vi "UIRef.vi"(8 "error in":errorcluster, 11 "PXI in":refnum<class "PLTarget PXI.lvclass">) -> (0 "error out":errorcluster, 2 "VI refnum":refnum<vi>, 3 "PXI out":refnum<class "PLTarget PXI.lvclass">)   [LabVIEW 2013, in "PLTarget PXI.lvclass"]
uses:
  PLTarget PXI.lvclass
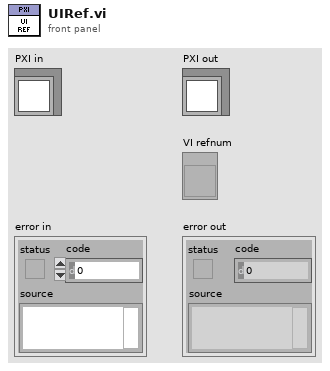
[diagram p1: front panel]
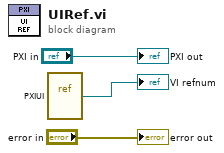
[diagram p0: block diagram]
diagram:
  n1 = vi-ref "PXIUI.vi"() -> (→"VI refnum":refnum<vi>)
  "error out" <- "error in"
  "PXI out" <- "PXI in"
